vi "1-1.vi"() -> ()   [LabVIEW 2022 SP3, in "AoC22.lvlib"]
uses:
  AoC22.lvlib
panel:
  out "max value":i32
  out "string array":string[](array[string])
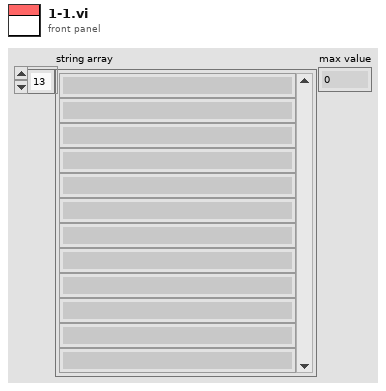
[diagram p1: front panel]
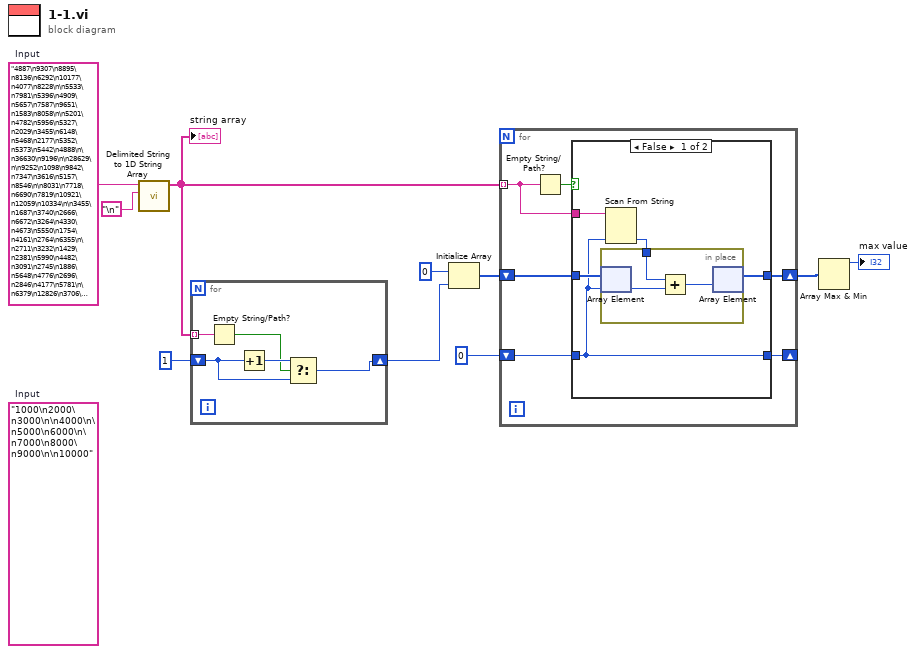
[diagram p0: block diagram]
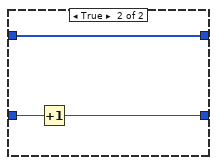
[diagram p2: hidden frame]
diagram:
  (unwired) "1000\n2000\n3000\n\n4000\n\n5000\n6000\n\n7000\n8000\n9000\n\n10000"  # Input
  w8 = "4887\n9307\n8895\n8136\n6292\n10177\n4077\n8228\n\n5533\n7981\n5396\n4909\n5657\n7587\n9651\n1583\n8058\n\n5201\n4782\n5956\n5327\n2029\n3455\n6148\n5468\n2177\n5352\n5373\n5442\n4888\n\n36630\n9196\n\n28629\n\n9252\n1098\n9842\n7347\n3616\n5157\n8546\n\n8031\n7718\n6690\n7819\n10921\n12059\n10334\n\n3455\n1687\n3740\n2666\n6672\n3264\n4330\n4673\n5550\n1754\n4161\n2764\n6355\n\n2711\n3232\n1429\n2381\n5990\n4482\n3091\n2745\n1886\n5648\n4776\n2696\n2846\n4177\n5781\n\n6379\n12826\n3706\n12650\n5875\n11396\n\n10381\n2204\n5950\n11465\n11501\n13306\n\n4006\n6635\n5139\n5290\n4562\n5558\n2788\n1242\n5308\n6704\n6858\n3751\n\n3574\n5601\n4492\n4795\n2135\n3295\n6150\n4786\n6761\n5098\n6646\n5839\n1989\n\n14468\n13500\n11..."  # Input
  n1 = call <vilib>:"Delimited String to 1D String Array.vi"("delimiter"="\n", "delimited string"=w8) -> ("string array"=w5:string[])  [unwired: 9 in]
  "string array" <- w5
  n2 = for {
    tunnel: w5 -> [w15] mode=indexing
    shift-right: [w14] -> w7
    shift-left: 1 -> [w13]
    n3 = Empty String/Path?(string/path=w15) -> (empty?=w11:bool)
    n4 = Increment(x=w13) -> (x+1=w12:i32)
    n5 = Select(t=w12, s=w11, f=w13) -> (s? t:f=w14:i32)
  }
  n6 = Initialize Array(0 ("element"), w7) -> (w4:i32[])
  n7 = for {
    tunnel: w5 -> [w20] mode=indexing
    shift-right: [w16] -> w2
    shift-left: w4 -> [w18]
    shift-right: [w17] -> _
    shift-left: 0 -> [w19]
    n8 = Empty String/Path?(string/path=w20) -> (empty?=w21:bool)
    n9 = case shown="False" w21 {
      tunnel: w20 -> [w24 _]
      tunnel: w19 -> [w23 w32]
      tunnel: w18 -> [w26 w30]
      tunnel: [w23 w31] -> w17
      tunnel: [w25 w30] -> w16
      frame False {
        n10 = Scan From String(input string=w24, default 1=w23) -> (output 1=w22:i32)  [unwired: 3 in, 3 out]
        n11 = in-place {
          in-place-border: w22 -> [w27]
          n12 = in-place-array #1(w26, w23) -> (w29:i32)
          n13 = Add(x=w27, y=w29) -> (x+y=w28:i32)
          n14 = in-place-array #1(w28) -> (w25:i32[])  [unwired: 1 out]
        }
      }
      frame True {
        n15 = Increment(x=w32) -> (x+1=w31:i32)
      }
    }
  }
  n16 = Array Max & Min(array=w2) -> (max value=→"max value":i32)  [unwired: 3 out]
